vi "EGSA.vi"() -> ()   [LabVIEW 2021]
panel:
  out "Array":string[](array[string])
  in  "stop":bool
  in  "Tab control":T1(tab)
  in  "?":bool
  in  "log in":bool
  in  "User Name":string
  in  "Password":string
  in  "Ground Track Track":bool
  in  "Determine Area":bool
  in  "Target determination":bool
  in  "Session Time":bool
  in  "Shadow and Light":bool
  in  "Satellite Position":bool
  in  "Track":bool
  in  "Orbiteal Elements":bool
  in  "Home":bool
  in  "Drop your path":path
  out "Satellite catalog number 2":string
  out "Inclination":string
  out "Right asciension of the ascending node":string
  out "Eccentricity":string
  out "Argument of perigee":string
  out "Mean anomaly":string
  out "Line number 2":string caption="Line number"
  out "Line number":string
  out "Satellite catalog number 1":string
  out "Last two digits Vof launch year":string
  out "Launch number of the year":string
  out "Epoch year":string
  out "Epoch day of year":string
  out "Classification":string caption="Line number"
  out "Piece of the launch":string
  out "Your TLE":string
  in  "?":bool
  in  "?":bool
  in  "Track Info":bool
  out "?":bool
  out "?":cluster{"X":dbl, "Y":dbl}[](graph)
  in  "?":bool
  out "Lat":dbl
  out "Long":i32
  out "V":string
  out "R":string
  in  "?":bool
  in  "?":bool
  in  "?":bool
  in  "?":bool
  in  "?":bool
  in  "?":bool
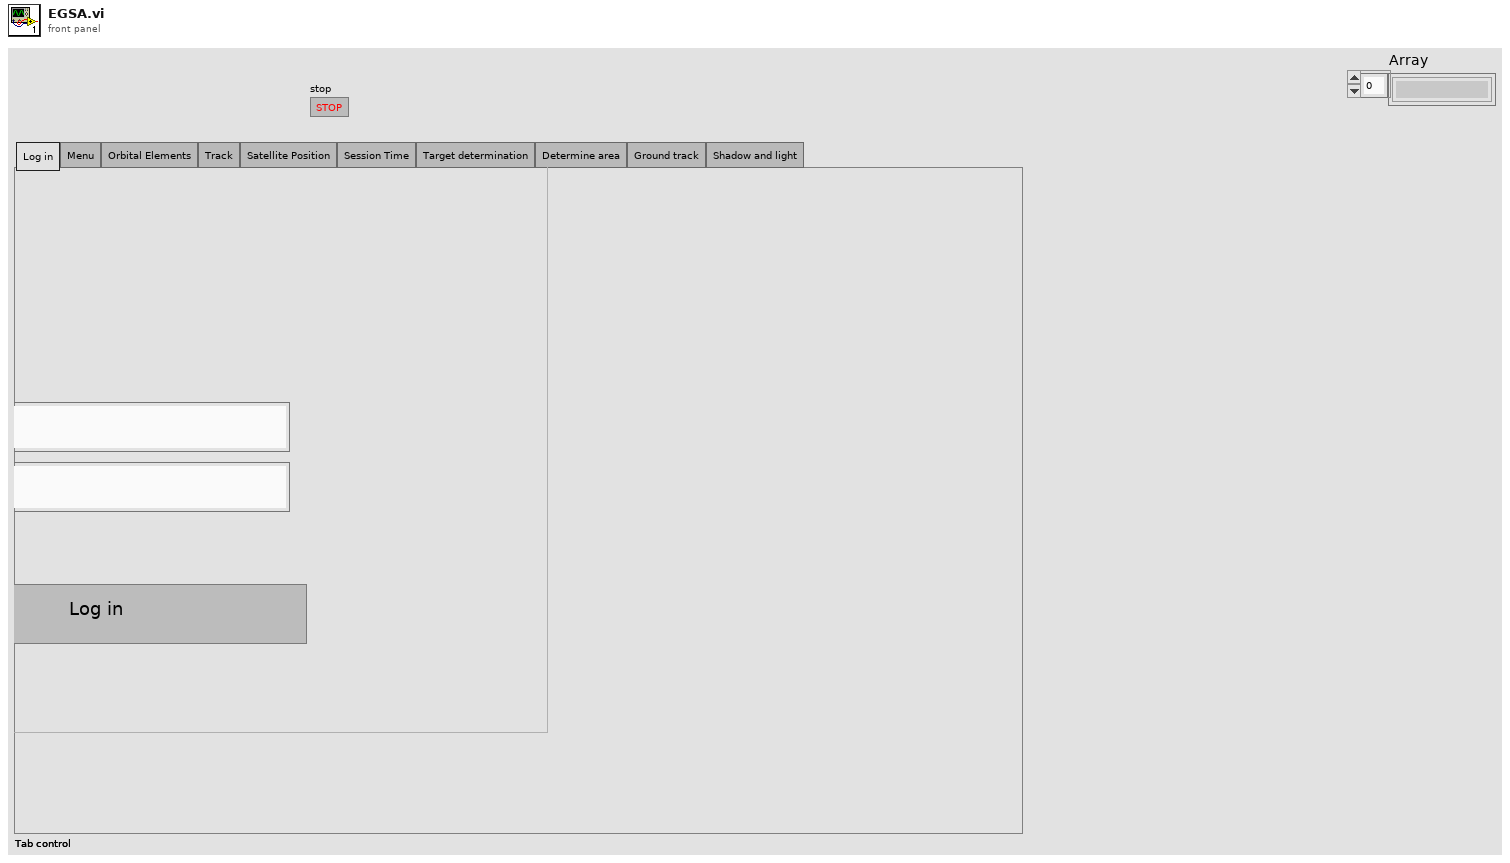
[diagram p1: front panel]
types:
  T1 = enum32{"Log in", "Menu", "Orbital Elements", "Track", "Satellite Position", "Session Time", "Target determination", "Determine area", "Ground track", "Shadow and light"}
  T2 = enum32{"Log in", "Menu", "Orbital Elements", "Track", "Satellite Position", "Session Time", "Target determination", "Determine area", "Ground track"}
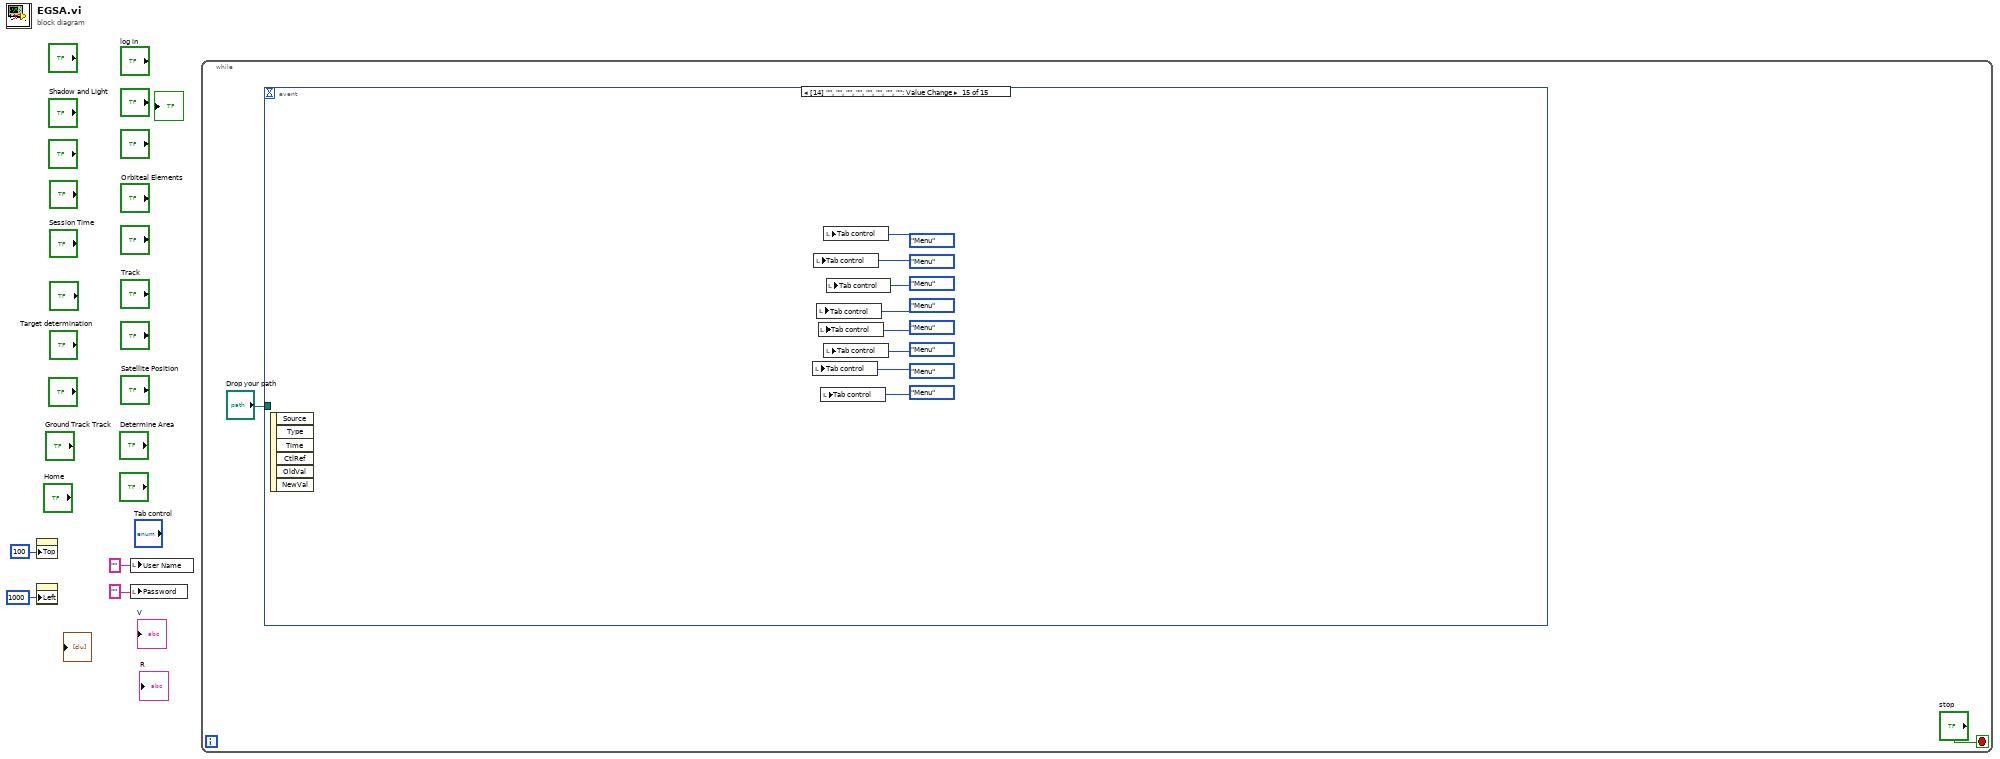
[diagram p0: block diagram]
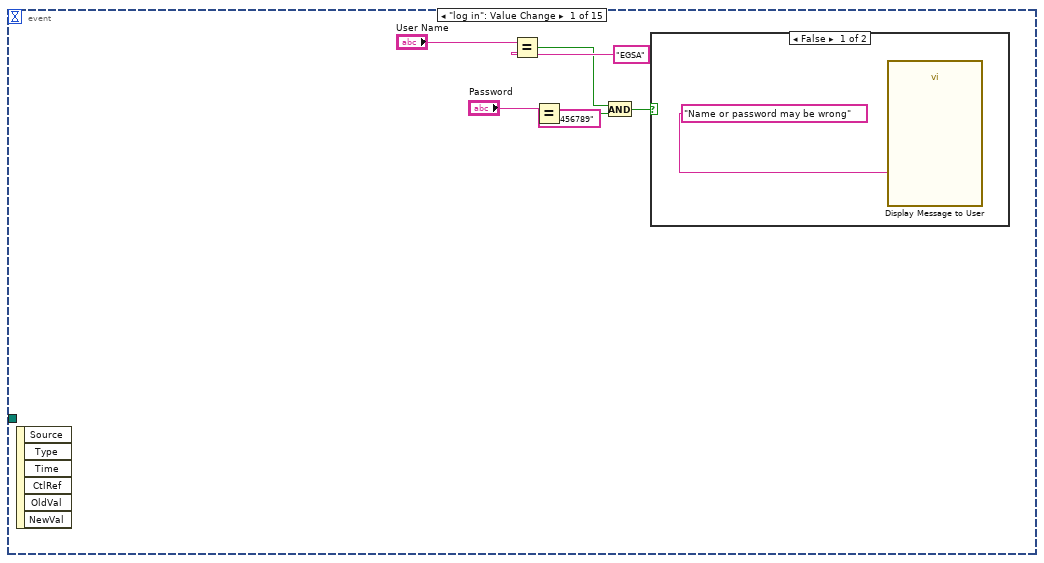
[diagram p2: hidden frame]
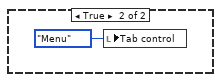
[diagram p3: hidden frame]
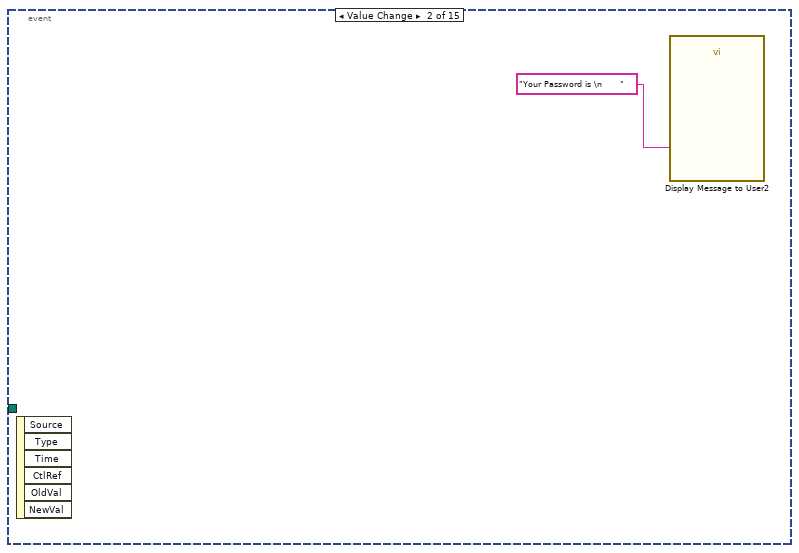
[diagram p4: hidden frame]
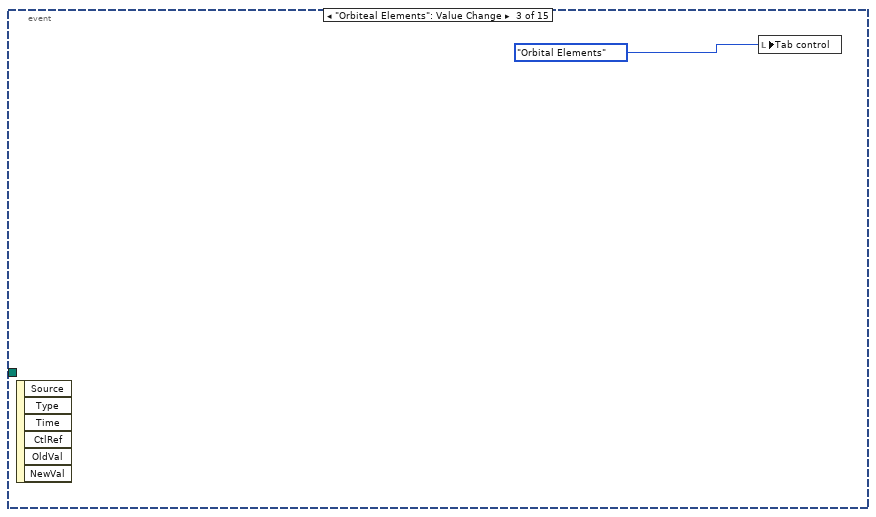
[diagram p5: hidden frame]
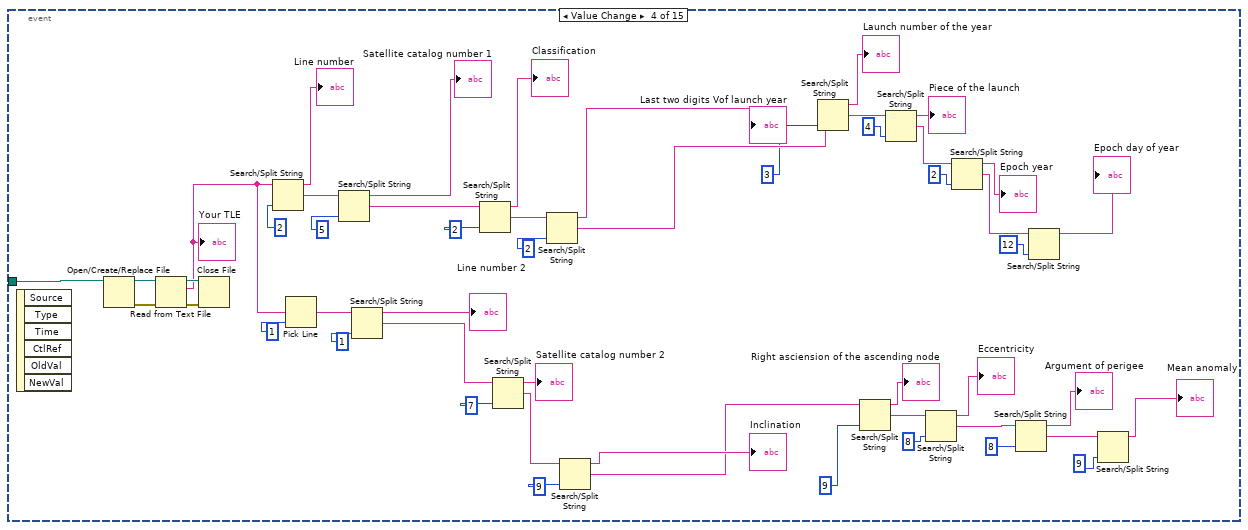
[diagram p6: hidden frame]
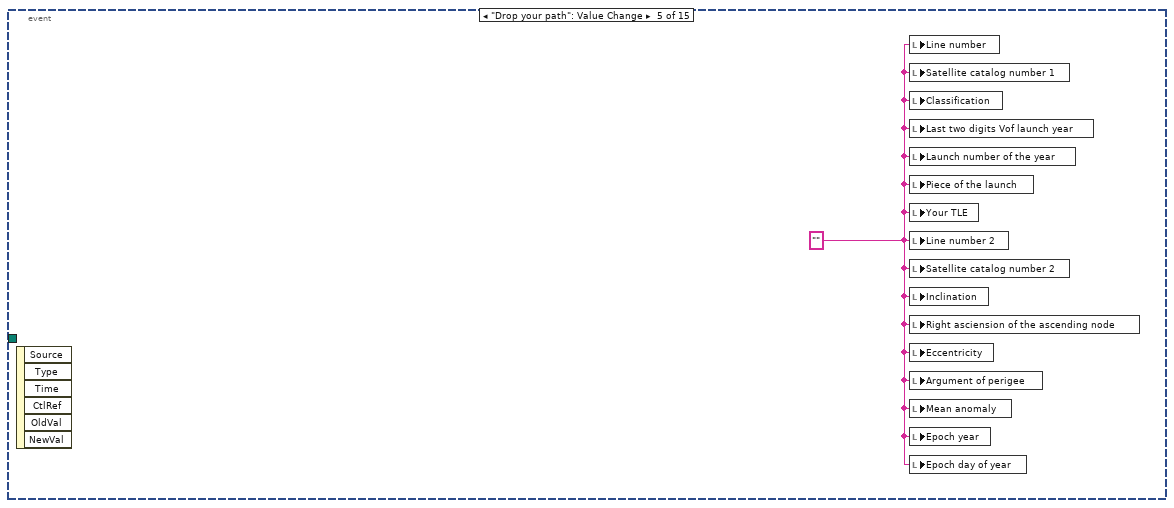
[diagram p7: hidden frame]
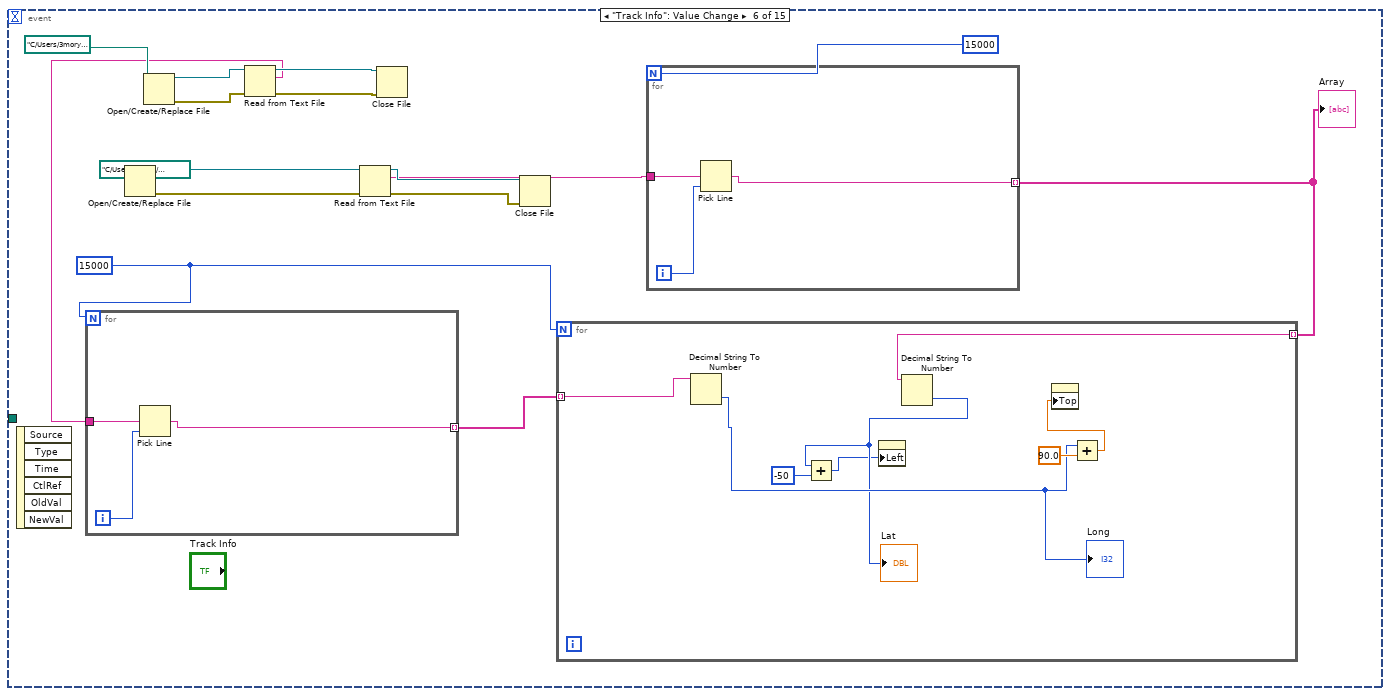
[diagram p8: hidden frame]
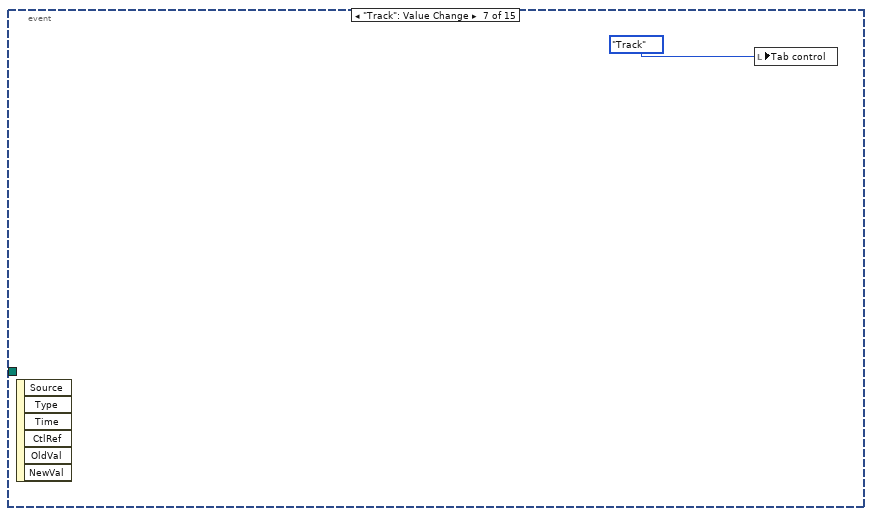
[diagram p9: hidden frame]
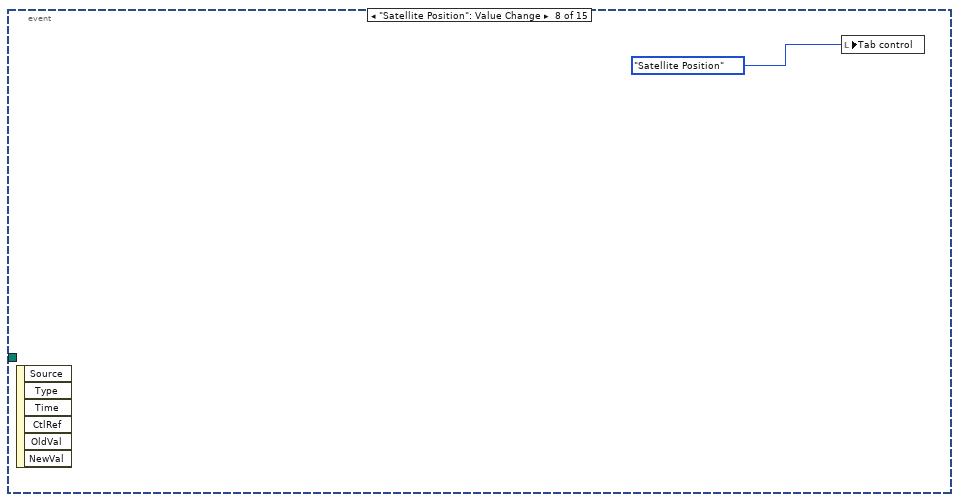
[diagram p10: hidden frame]
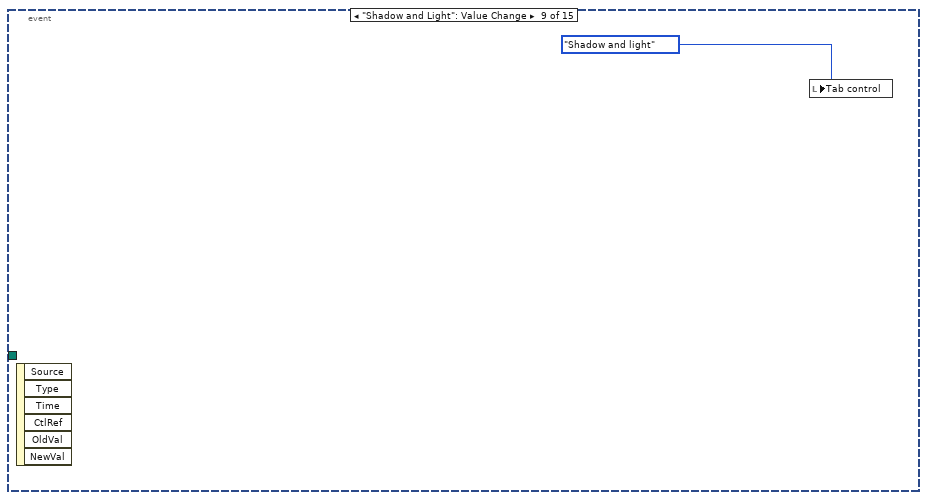
[diagram p11: hidden frame]
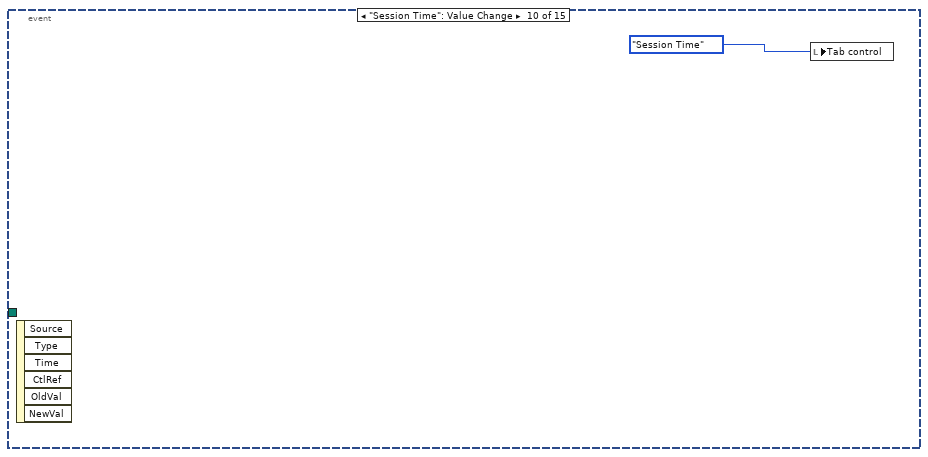
[diagram p12: hidden frame]
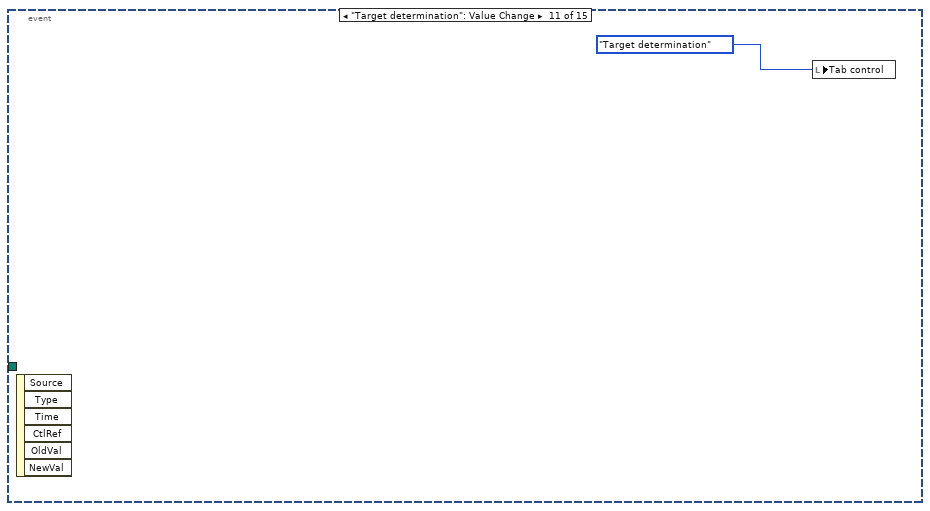
[diagram p13: hidden frame]
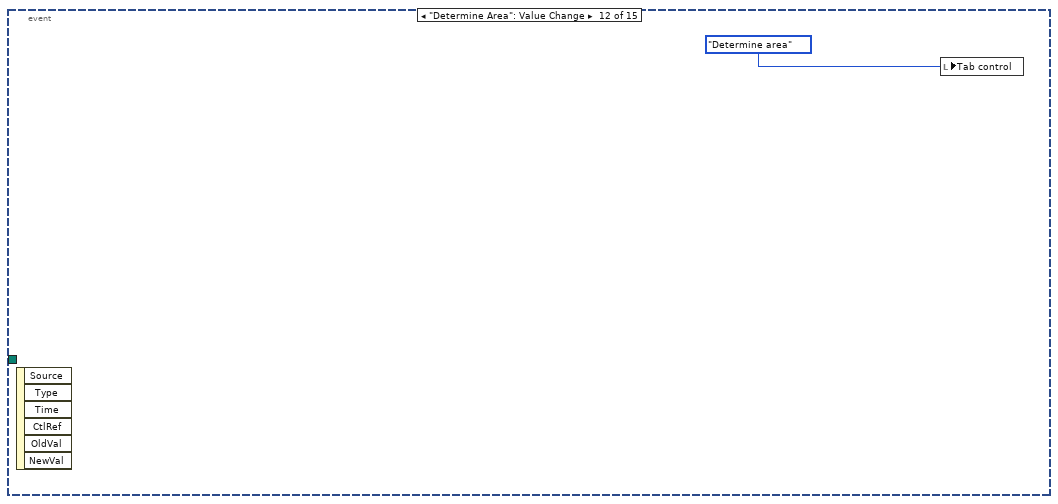
[diagram p14: hidden frame]
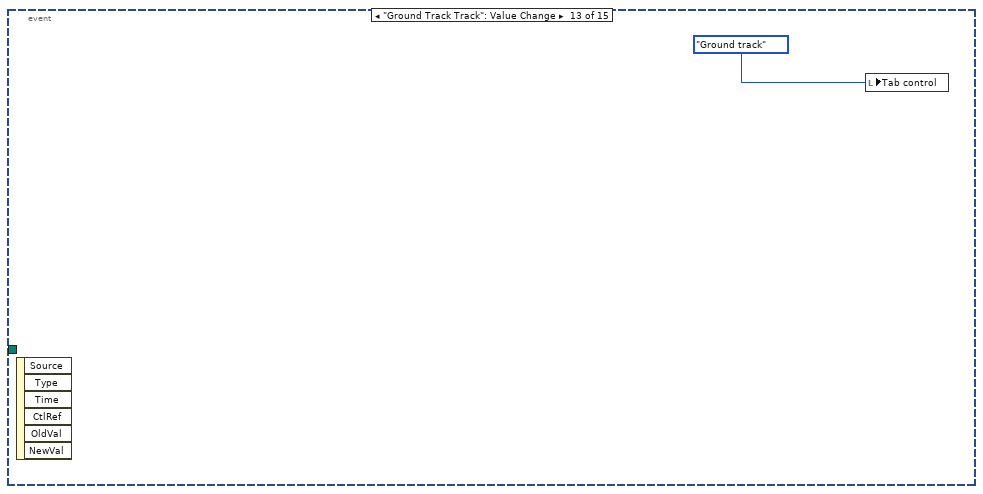
[diagram p15: hidden frame]
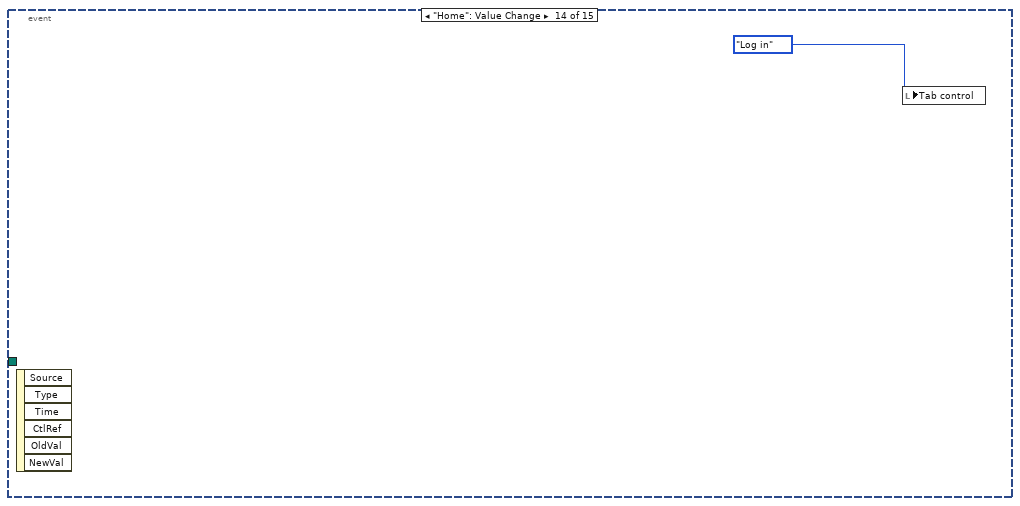
[diagram p16: hidden frame]
diagram:
  n1 = property class="Bool (strict)"("Top"=100 ("Position:Top")) -> ()  [unwired: 2 in, 2 out]
  n2 = property class="Bool (strict)"("Left"=1000 ("Position:Left")) -> ()  [unwired: 2 in, 2 out]
  n3 = local write "User Name"("" ("User Name")) -> ()
  n4 = local write "Password"("" ("Password")) -> ()
  n5 = while {
    stop <- "stop" stop-if-true
    n6 = event shown="[14] \"\", \"\", \"\", \"\", \"\", \"\", \"\", \"\": Value Change" {
      selector: _ -> [_ _ _ _ _ _ _ _ _ _ _ _ _ _ _]
      dyn-events: _ -> [_ _ _ _ _ _ _ _ _ _ _ _ _ _ _]
      timeout: _ -> [_ _ _ _ _ _ _ _ _ _ _ _ _ _ _]
      tunnel: "Drop your path" -> [_ _ _ w19 _ _ _ _ _ _ _ _ _ _ _]
      event "log in": Value Change {
        n7 = event-data() -> ()  [unwired: 1 in, 6 out]
        n8 = Equal?(x="User Name", y="EGSA") -> (x = y?=w8:bool)
        n9 = Equal?(x="Password", y="123456789") -> (x = y?=w9:bool)
        n10 = And(x=w8, y=w9) -> (x .and. y?=w7:bool)
        n11 = case shown="False" w7 {
          frame False {
            n12 = call "Display Message to User"("Message"="Name or password may be wrong") -> ()  [unwired: 9 in, 2 out]
          }
          frame True {
            n13 = local write "Tab control"(T1."Menu" ("Tab control")) -> ()
          }
        }
      }
      event Value Change {
        n14 = event-data() -> ()  [unwired: 1 in, 6 out]
        n15 = call "Display Message to User2"("Message"="Your Password is \n      ") -> ()  [unwired: 9 in, 2 out]
      }
      event "Orbiteal Elements": Value Change {
        n16 = event-data() -> ()  [unwired: 1 in, 6 out]
        n17 = local write "Tab control"(T1."Orbital Elements" ("Tab control")) -> ()
      }
      event Value Change {
        n18 = event-data() -> ()  [unwired: 1 in, 6 out]
        n19 = Open/Create/Replace File(file path (use dialog)=w19) -> (refnum out=w68:refnum<file>, error out=w67:errorcluster)  [unwired: 5 in, 1 out]
        n20 = Read from Text File(file (use dialog)=w68, error in=w67) -> (refnum out=w66:refnum<file>, text=w18:string, error out=w65:errorcluster)  [unwired: 2 in, 1 out]
        "Your TLE" <- w18
        n21 = Close File(refnum=w66, error in=w65) -> ()  [unwired: 2 out]
        n22 = Search/Split String(string=w18, offset (0)=2) -> (substring before match=→"Line number":string, match + rest of string=w35:string)  [unwired: 1 in, 1 out]
        n23 = Pick Line(multi-line string=w18, line index=1) -> (output string=w20:string)  [unwired: 1 in]
        n24 = Search/Split String(string=w35, offset (0)=5) -> (substring before match=→"Satellite catalog number 1":string, match + rest of string=w25:string)  [unwired: 1 in, 1 out]
        n25 = Search/Split String(string=w20, offset (0)=1) -> (substring before match=→"Line number 2":string, match + rest of string=w48:string)  [unwired: 1 in, 1 out]
        n26 = Search/Split String(string=w25, offset (0)=2) -> (substring before match=→"Classification":string, match + rest of string=w27:string)  [unwired: 1 in, 1 out]
        n27 = Search/Split String(string=w48, offset (0)=7) -> (substring before match=→"Satellite catalog number 2":string, match + rest of string=w46:string)  [unwired: 1 in, 1 out]
        n28 = Search/Split String(string=w27, offset (0)=2) -> (substring before match=→"Last two digits Vof launch year":string, match + rest of string=w32:string)  [unwired: 1 in, 1 out]
        n29 = Search/Split String(string=w46, offset (0)=9) -> (substring before match=→"Inclination":string, match + rest of string=w44:string)  [unwired: 1 in, 1 out]
        n30 = Search/Split String(string=w32, offset (0)=3) -> (substring before match=→"Launch number of the year":string, match + rest of string=w24:string)  [unwired: 1 in, 1 out]
        n31 = Search/Split String(string=w44, offset (0)=9) -> (substring before match=→"Right asciension of the ascending node":string, match + rest of string=w42:string)  [unwired: 1 in, 1 out]
        n32 = Search/Split String(string=w24, offset (0)=4) -> (substring before match=→"Piece of the launch":string, match + rest of string=w23:string)  [unwired: 1 in, 1 out]
        n33 = Search/Split String(string=w42, offset (0)=8) -> (substring before match=→"Eccentricity":string, match + rest of string=w40:string)  [unwired: 1 in, 1 out]
        n34 = Search/Split String(string=w23, offset (0)=2) -> (substring before match=→"Epoch year":string, match + rest of string=w30:string)  [unwired: 1 in, 1 out]
        n35 = Search/Split String(string=w40, offset (0)=8) -> (substring before match=→"Argument of perigee":string, match + rest of string=w38:string)  [unwired: 1 in, 1 out]
        n36 = Search/Split String(string=w30, offset (0)=12) -> (substring before match=→"Epoch day of year":string)  [unwired: 1 in, 2 out]
        n37 = Search/Split String(string=w38, offset (0)=9) -> (substring before match=→"Mean anomaly":string)  [unwired: 1 in, 2 out]
      }
      event "Drop your path": Value Change {
        w69 = "" ("Line number")
        n38 = event-data() -> ()  [unwired: 1 in, 6 out]
        n39 = local write "Line number"(w69) -> ()
        n40 = local write "Satellite catalog number 1"(w69) -> ()
        n41 = local write "Classification"(w69) -> ()
        n42 = local write "Last two digits Vof launch year"(w69) -> ()
        n43 = local write "Launch number of the year"(w69) -> ()
        n44 = local write "Piece of the launch"(w69) -> ()
        n45 = local write "Your TLE"(w69) -> ()
        n46 = local write "Line number 2"(w69) -> ()
        n47 = local write "Satellite catalog number 2"(w69) -> ()
        n48 = local write "Inclination"(w69) -> ()
        n49 = local write "Right asciension of the ascending node"(w69) -> ()
        n50 = local write "Eccentricity"(w69) -> ()
        n51 = local write "Argument of perigee"(w69) -> ()
        n52 = local write "Mean anomaly"(w69) -> ()
        n53 = local write "Epoch year"(w69) -> ()
        n54 = local write "Epoch day of year"(w69) -> ()
      }
      event "Track Info": Value Change {
        w70 = 15000
        n55 = event-data() -> ()  [unwired: 1 in, 6 out]
        n56 = Open/Create/Replace File(file path (use dialog)=path "C:/Users/3mory/OneDrive - Beni-suef University (Beni-suef University)/Desktop/Long.txt") -> (refnum out=w85:refnum<file>, error out=w84:errorcluster)  [unwired: 5 in, 1 out]
        n57 = Open/Create/Replace File(file path (use dialog)=path "C:/Users/3mory/OneDrive - Beni-suef University (Beni-suef University)/Desktop/Lat.txt") -> (refnum out=w81:refnum<file>, error out=w80:errorcluster)  [unwired: 5 in, 1 out]
        n58 = Read from Text File(file (use dialog)=w81, error in=w80) -> (refnum out=w79:refnum<file>, text=w72:string, error out=w78:errorcluster)  [unwired: 2 in, 1 out]
        n59 = for {
          N: w70 -> [_]
          tunnel: w72 -> [w87]
          tunnel: [w86] -> w71 mode=indexing
          i -> [w88]
          n60 = Pick Line(multi-line string=w87, line index=w88) -> (output string=w86:string)  [unwired: 1 in]
        }
        n61 = Read from Text File(file (use dialog)=w85, error in=w84) -> (refnum out=w83:refnum<file>, text=w75:string, error out=w82:errorcluster)  [unwired: 2 in, 1 out]
        n62 = Close File(refnum=w79, error in=w78) -> ()  [unwired: 2 out]
        n63 = Close File(refnum=w83, error in=w82) -> ()  [unwired: 2 out]
        n64 = for {
          N: 15000 -> [_]
          tunnel: w75 -> [w98]
          tunnel: [w97] -> w73 mode=indexing
          i -> [w99]
          n65 = Pick Line(multi-line string=w98, line index=w99) -> (output string=w97:string)  [unwired: 1 in]
        }
        "Array" <- w73
        n66 = for {
          N: w70 -> [_]
          tunnel: w73 -> [w96] mode=indexing
          tunnel: w71 -> [w95] mode=indexing
          n67 = Decimal String To Number(string=w95) -> (number=w93:i32)  [unwired: 2 in, 1 out]
          "Long" <- w93
          n68 = Decimal String To Number(string=w96) -> (number=w91:i32)  [unwired: 2 in, 1 out]
          "Lat" <- w91
          n69 = Add(x=w91, y=-50) -> (x+y=w89:i32)
          n70 = property class="Bool (strict)"("Left"=w89) -> ()  [unwired: 2 in, 2 out]
          n71 = Add(x=w93, y=90.0) -> (x+y=w92:dbl)
          n72 = property class="Bool (strict)"("Top"=w92) -> ()  [unwired: 2 in, 2 out]
        }
      }
      event "Track": Value Change {
        n73 = event-data() -> ()  [unwired: 1 in, 6 out]
        n74 = local write "Tab control"(T1."Track" ("Tab control")) -> ()
      }
      event "Satellite Position": Value Change {
        n75 = event-data() -> ()  [unwired: 1 in, 6 out]
        n76 = local write "Tab control"(T2."Satellite Position" ("Tab control")) -> ()
      }
      event "Shadow and Light": Value Change {
        n77 = event-data() -> ()  [unwired: 1 in, 6 out]
        n78 = local write "Tab control"(T1."Shadow and light" ("Tab control")) -> ()
      }
      event "Session Time": Value Change {
        n79 = event-data() -> ()  [unwired: 1 in, 6 out]
        n80 = local write "Tab control"(T1."Session Time" ("Tab control")) -> ()
      }
      event "Target determination": Value Change {
        n81 = event-data() -> ()  [unwired: 1 in, 6 out]
        n82 = local write "Tab control"(T1."Target determination" ("Tab control")) -> ()
      }
      event "Determine Area": Value Change {
        n83 = event-data() -> ()  [unwired: 1 in, 6 out]
        n84 = local write "Tab control"(T1."Determine area" ("Tab control")) -> ()
      }
      event "Ground Track Track": Value Change {
        n85 = event-data() -> ()  [unwired: 1 in, 6 out]
        n86 = local write "Tab control"(T1."Ground track" ("Tab control")) -> ()
      }
      event "Home": Value Change {
        n87 = event-data() -> ()  [unwired: 1 in, 6 out]
        n88 = local write "Tab control"(T1."Log in" ("Tab control")) -> ()
      }
      event Value Change {
        n89 = event-data() -> ()  [unwired: 1 in, 6 out]
        n90 = local write "Tab control"(T1."Menu" ("Tab control")) -> ()
        n91 = local write "Tab control"(T1."Menu" ("Tab control")) -> ()
        n92 = local write "Tab control"(T1."Menu" ("Tab control")) -> ()
        n93 = local write "Tab control"(T1."Menu" ("Tab control")) -> ()
        n94 = local write "Tab control"(T1."Menu" ("Tab control")) -> ()
        n95 = local write "Tab control"(T1."Menu" ("Tab control")) -> ()
        n96 = local write "Tab control"(T1."Menu" ("Tab control")) -> ()
        n97 = local write "Tab control"(T1."Menu" ("Tab control")) -> ()
      }
    }
  }
